vi "Destroy.vi"(8 "error in (no error)":errorcluster, 10 "RT_Game.lvlib:Engine.lvclass":refnum<class "Engine.lvclass">, 11 "SnakeGame in":refnum<class "SnakeGame.lvclass">) -> (0 "error out":errorcluster, 2 "RT_Game.lvlib:Engine.lvclass 2":refnum<class "Engine.lvclass">, 3 "FPGA_ref":T1)   [LabVIEW 2019, in "RT_Game.lvlib" / "SnakeGame.lvclass"]
uses:
  SnakeGame.lvclass
  FPGA_Interface.ctl
  Engine/Engine.lvclass
  Game/Game.lvclass
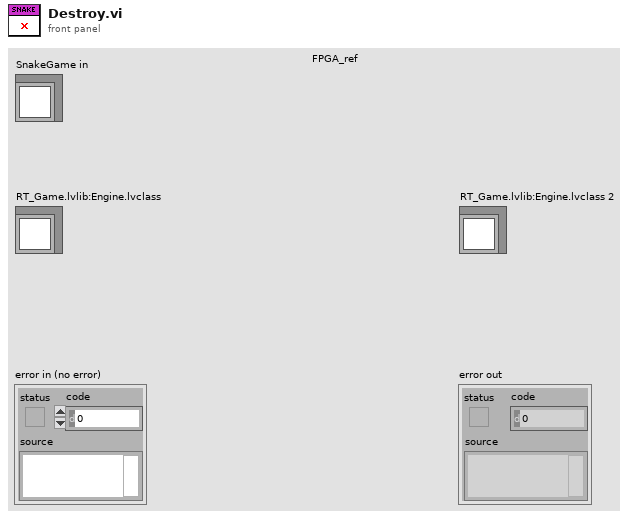
[diagram p1: front panel]
types:
  T1 = typedef "FPGA_Interface.ctl" = refnum<k20>
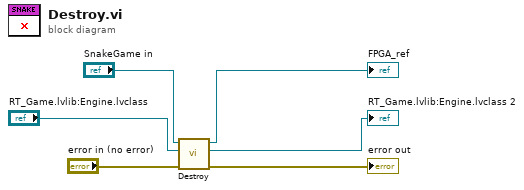
[diagram p0: block diagram]
diagram:
  n1 = call-parent "Destroy.vi"("error in (no error)"="error in (no error)", "RT_Game.lvlib:Engine.lvclass"="RT_Game.lvlib:Engine.lvclass", "Game in"="SnakeGame in") -> ("error out"=→"error out":errorcluster, "RT_Game.lvlib:Engine.lvclass 2"=→"RT_Game.lvlib:Engine.lvclass 2":refnum<class "Engine.lvclass">, "FPGA_ref"=→"FPGA_ref":T1)  [unwired: 6 in]
